vi "Revision Query.vi"(8 "error in (no error)":errorcluster {"code" format="%.0x"}, 11 "instrument handle":refnum<k15>) -> (0 "error out":errorcluster {"code" format="%.0x"}, 1 "firmware revision":string, 2 "instrument driver revision":string, 3 "instrument handle out":refnum<k15>)   [LabVIEW 2014, in "Agilent NA.lvlib"]
doc: "Retrieves revision information from the instrument."
uses:
  Agilent NA.lvlib
  AgNA.dll
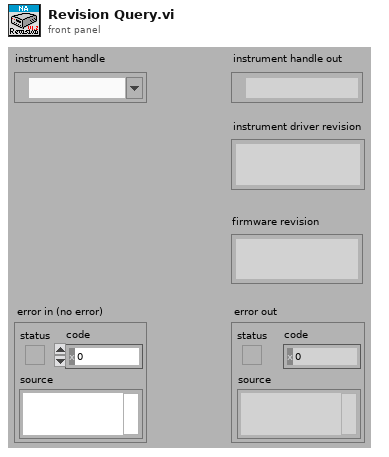
[diagram p1: front panel]
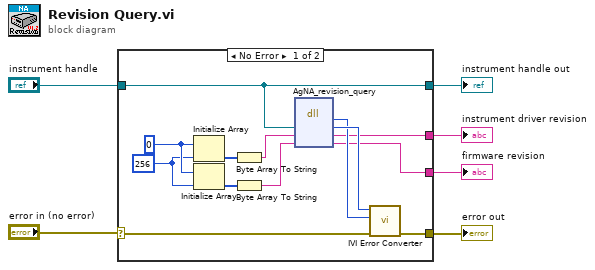
[diagram p0: block diagram]
diagram:
  n1 = case shown="No Error" "error in (no error)" {
    selector: "error in (no error)" -> [w10 w20]
    tunnel: [w9 w21] -> w5
    tunnel: "instrument handle" -> [w9 w21]
    tunnel: [w14 w20] -> w3
    tunnel: [w8 _] -> w2
    tunnel: [w7 _] -> w1
    frame No Error {
      w11 = 256
      w12 = u8 0
      n2 = Initialize Array(w12, w11) -> (w19:u8[])
      n3 = Initialize Array(w12, w11) -> (w18:u8[])
      n4 = Byte Array To String(unsigned byte array=w19) -> (string=w17:string)
      n5 = Byte Array To String(unsigned byte array=w18) -> (string=w16:string)
      n6 = dll-call lib="AgNA**.dll" fn="AgNA_revision_query" ("LabVIEW:IviDmm_revision_query")("instrument handle"=w9, "instrument driver revision"=w17, "firmware revision"=w16) -> ("Status"=w13:i32, "instrument handle"=w15:u32, "instrument driver revision"=w7:string, "firmware revision"=w8:string)  [unwired: 3 in, 2 out]
      n7 = call "IVI Error Converter.vi"("error in (no error)"=w10, "IVI error code (0)"=w13, "instrument handle"=w15) -> ("error out"=w14:errorcluster)  [unwired: 7 in, 1 out]
    }
    frame Error {
    }
  }
  "error out" <- w3
  "instrument handle out" <- w5
  "instrument driver revision" <- w1
  "firmware revision" <- w2
